vi "Execute.vi"(8 "error in":errorcluster, 11 "O3 Generator Power STEP in":refnum<class "O3 Generator Power STEP.lvclass">) -> (0 "error out":errorcluster, 1 "Next Step?":bool, 2 "MSG":string, 3 "O3 Generator Power STEP out":refnum<class "O3 Generator Power STEP.lvclass">)   [LabVIEW 2014, in "O3 Generator Power STEP.lvclass"]
uses:
  O3 Generator Power STEP.lvclass
  <vilib>/ActorFramework/Message Enqueuer/Message Enqueuer.lvclass
  Controller/Messages/Change Individual Power Supply State/Change Individual Power Supply MSG.lvclass
  reusable/Sequence/STEPS/STEP.lvclass/STEP.ctl
  Controller/Messages/Change Individual Power Supply State/Change Individual Power Supply MSG.lvclass/Change Individual Power Supply MSG.ctl
  <vilib>/ActorFramework/Message Enqueuer/Message Enqueuer.lvclass/Message Enqueuer.ctl
  reusable/Sequence/STEPS/Read Obj.vi
  Controller/Messages/Change Individual Power Supply State/Write Index.vi
  Controller/Messages/Change Individual Power Supply State/Write State.vi
  <vilib>/ActorFramework/Message Priority Queue/Priority Enqueue.vi
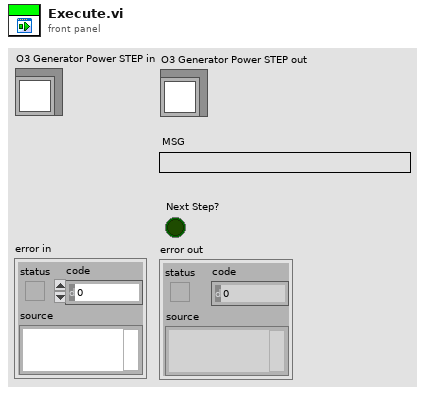
[diagram p1: front panel]
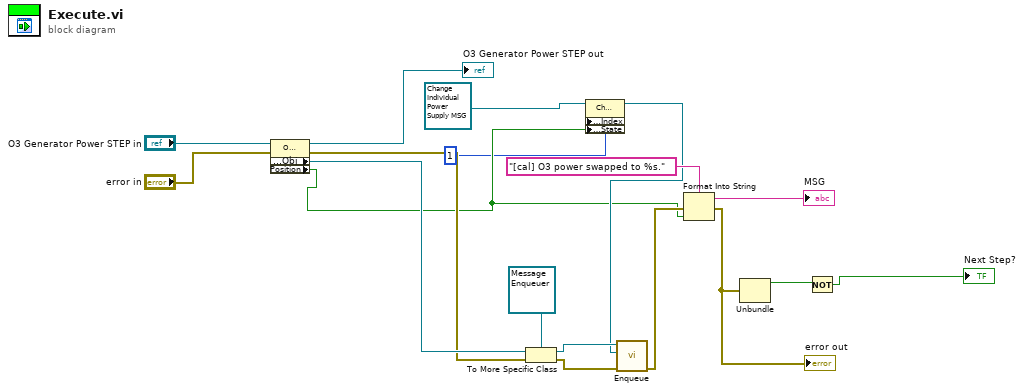
[diagram p0: block diagram]
diagram:
  n1 = property class="O3 Generator Power"(reference="O3 Generator Power STEP in", error in="error in") -> (reference out=→"O3 Generator Power STEP out":refnum<class "O3 Generator Power STEP.lvclass">, error out=w14:errorcluster, "Accessors:Obj"=w17:refnum<class>, "Position"=w2:bool)
  n2 = To More Specific Class(target class=refnum<class "Message Enqueuer.lvclass"> refnum ("Message Enqueuer in"), reference=w17, error in=w14) -> (specific class reference=w12:refnum<class "Message Enqueuer.lvclass">, error out=w13:errorcluster)
  n3 = property class="Change Individual Power Supply"(reference=refnum<class "Change Individual Power Supply MSG.lvclass"> refnum ("Controller:Change Individual Power Supply"), "Accessors:Index"=1 ("Index"), "Accessors:State"=w2) -> (reference out=w4:refnum<class "Change Individual Power Supply MSG.lvclass">)  [unwired: 1 in, 1 out]
  n4 = call <vilib>:"Enqueue.vi"("error in (no error)"=w13, "Message"=w4, "Message Enqueuer in"=w12) -> ("error out"=w9:errorcluster)  [unwired: 7 in, 1 out]
  n5 = Format Into String(format string="[cal] O3 power swapped to %s.", error in=w9, w2) -> (resulting string=→"MSG":string, error out=w8:errorcluster)  [unwired: 1 in]
  "error out" <- w8
  n6 = Unbundle(w8) -> ("status"=w7:bool)  [unwired: 2 out]
  n7 = Not(x=w7) -> (.not. x?=→"Next Step?":bool)
